vi "OscilControl.vi"() -> ()   [LabVIEW 2024]
panel:
  out "concatenated string":string
  out "data out":string
  in  "Channel":string="1"
  in  "Combo Box":string(combo)
  in  "address":string
  out "error out":errorcluster
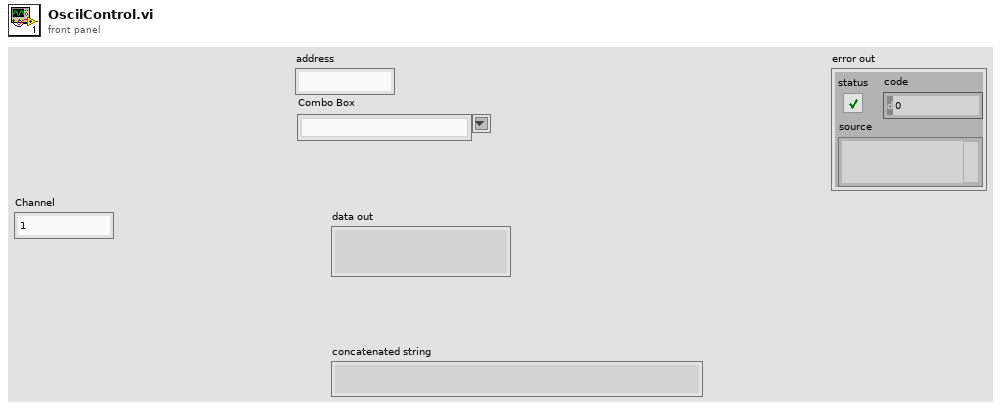
[diagram p1: front panel]
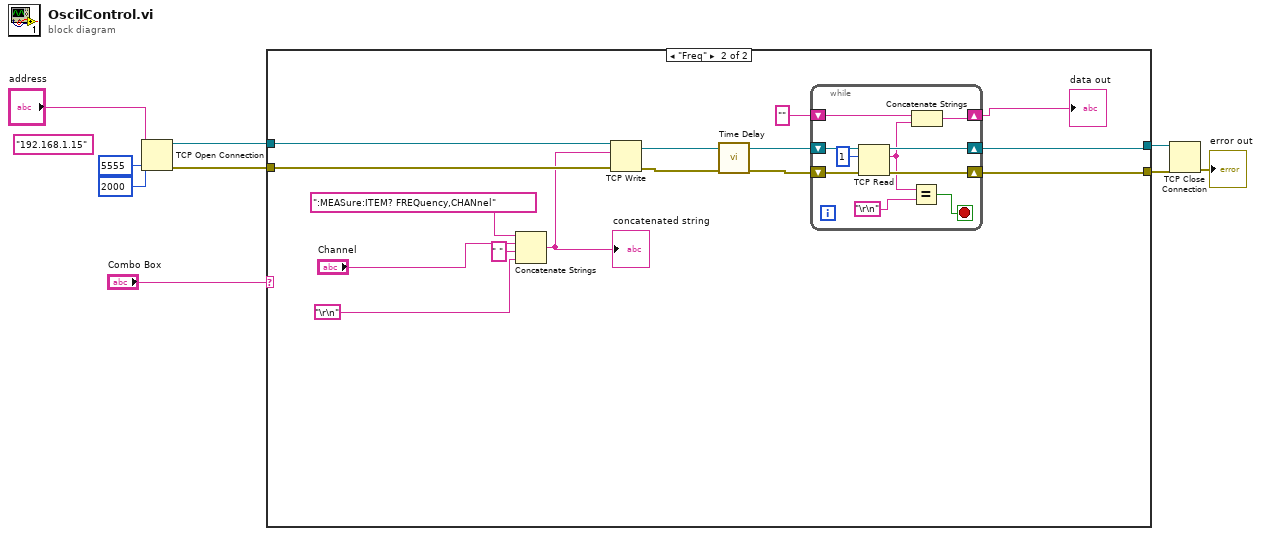
[diagram p0: block diagram]
diagram:
  (unwired) "192.168.1.15" ("address")
  n1 = TCP Open Connection(address="address", remote port or service name=u16 5555, timeout ms (60000)=2000) -> (connection ID=w9:refnum<k5>, error out=w8:errorcluster)  [unwired: 2 in]
  n2 = case shown="\"Freq\"" "Combo Box" {
    tunnel: w9 -> [w11 w25]
    tunnel: w8 -> [w10 w24]
    tunnel: [w11 w19] -> w6
    tunnel: [w10 w18] -> w5
    frame "Duty", Default {
    }
    frame "Freq" {
      n3 = Concatenate Strings(":MEASure:ITEM? FREQuency,CHANnel", "Channel", " " ("string"), "\r\n") -> (w22:string)
      "concatenated string" <- w22
      n4 = TCP Write(connection ID=w25, data in=w22, error in (no error)=w24) -> (connection ID out=w20:refnum<k5>, error out=w15:errorcluster)  [unwired: 1 in, 1 out]
      n5 = call "Time Delay"("error in (no error)"=w15) -> ("error out"=w14:errorcluster)  [unwired: 10 in]
      n6 = while {
        shift-right: [w34] -> w19
        shift-left: w20 -> [w35]
        shift-right: [w33] -> w18
        shift-left: w14 -> [w31]
        shift-right: [w29] -> w12
        shift-left: "" ("data out") -> [w30]
        stop <- w26 stop-if-true
        n7 = TCP Read(connection ID=w35, bytes to read=1, error in (no error)=w31) -> (connection ID out=w34:refnum<k5>, data out=w28:string, error out=w33:errorcluster)  [unwired: 2 in]
        n8 = Equal?(x=w28, y="\r\n") -> (x = y?=w26:bool)
        n9 = Concatenate Strings(w30, w28) -> (w29:string)
      }
      "data out" <- w12
    }
  }
  n10 = TCP Close Connection(connection ID=w6, error in (no error)=w5) -> (error out=→"error out":errorcluster)  [unwired: 1 in, 1 out]
